vi "Measure File Load Duration.vi"(11 "path":path) -> (3 "duration":dbl format="%.3f s")   [LabVIEW 2017, in "DSF Core.lvlib" / "Configuration Session.lvclass"]
uses:
  Classes/Configuration/Configuration Session.lvclass
  <vilib>/Platform/TimedLoop/XDataNode/timing_clust.ctl
  <vilib>/Platform/TimedLoop/XDataNode/nitl_modes.ctl
  <vilib>/Platform/TimedLoop/XDataNode/wakeup.ctl
  <vilib>/platform/TimedLoop/XDataNode/XDataNode.xnode
  <vilib>/Platform/TimedLoop/XDataNode/XDNodeRunTimeDep.lvlib
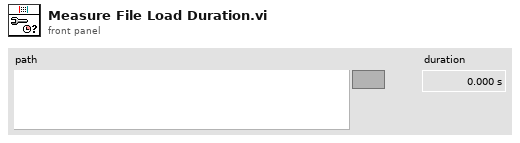
[diagram p1: front panel]
types:
  T1 = typedef "XDNodeRunTimeDep.lvlib/timing_clust.ctl" = cluster{"Expected End [f-1]":u64, "Actual End [f-1]":u64, "Finished Late? [f-1]":bool, "Expected End [i-1]":u64, "Actual End [i-1]":u64, "Finished Late? [i-1]":bool, "Expected Start [i]":u64, "Actual Start [i]":u64, "Expected Start [f]":u64, "Actual Start [f]":u64, "Source Name":string, "Structure Name":string, "Period":i64, "Deadline":i64, "Offset":i64, "Start":i64, "Priority":i32, "Timeout":i32, "Mode":T2, "Wakeup Reason":T3, "Error":errorcluster, "Source Type":string, "Secondary Source Type":string, "Global End Time":u64, "Global Start Time":u64, "Frame Duration":u64, "Iteration Duration":u64, "Assigned CPU":i32, "I/O Scan Engine Mode":u32}
  T2 = typedef "XDNodeRunTimeDep.lvlib/nitl_modes.ctl" = enum32{"No Change", "Process missed periods, maintain original phase", "Discard missed periods, maintain original phase", "Process missed periods, ignore original phase", "Discard missed periods, ignore original phase"}
  T3 = typedef "XDNodeRunTimeDep.lvlib/wakeup.ctl" = enum32{"Normal", "Aborted", "Asynchronous wakeup", "Timing source error", "Timed loop error", "Timeout"}
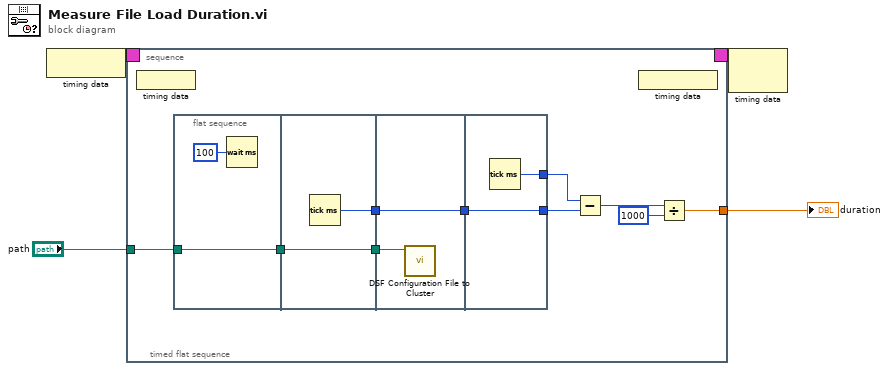
[diagram p0: block diagram]
diagram:
  n1 = node-c288() -> (w3:T1)
  n2 = timed-sequence {
    timing: w3 -> [_]
    timing-out: [_] -> w2
    tunnel: "path" -> [w6]
    tunnel: [w5] -> w1
    n3 = timed-flat-sequence {
      tunnel: w6 -> [w12]
      tunnel: [w7] -> w5
      n4 = node-c288() -> ()  [unwired: 1 in]
      n5 = flat-sequence {
        tunnel: w12 -> [w18]
        tunnel: [w18] -> w16
        tunnel: w16 -> [w20]
        tunnel: [w20] -> w15
        tunnel: [w19] -> w14
        tunnel: w15 -> [w21]
        tunnel: w14 -> [w22]
        tunnel: [w22] -> w13
        tunnel: w13 -> [w24]
        tunnel: [w24] -> w11
        tunnel: [w23] -> w10
        frame #0 {
          n6 = Wait (ms)(milliseconds to wait=u32 100) -> ()  [unwired: 1 out]
        }
        frame #1 {
          n7 = Tick Count (ms)() -> (millisecond timer value=w19:u32)
        }
        frame #2 {
          n8 = call "DSF Configuration File to Cluster.vi"("dsf configuration file path"=w21) -> ()  [unwired: 8 in, 3 out]
        }
        frame #3 {
          n9 = Tick Count (ms)() -> (millisecond timer value=w23:u32)
        }
      }
      n10 = Subtract(x=w10, y=w11) -> (x-y=w9:u32)
      n11 = node-c288() -> ()  [unwired: 1 out]
      n12 = Divide(x=w9, y=u32 1000) -> (x/y=w7:dbl)
    }
  }
  "duration" <- w1
  n13 = node-c288(w2) -> ()  [unwired: 1 out]
